vi "TxChannel - Get Tx Channels.vi"(7 "MCLB":refnum<vi>, 8 "error in (no error)":errorcluster, 11 "Node Ptr":T1 format="%.0x") -> (0 "error out":errorcluster, 3 "Node Ptr out":T1 format="%.0x", 5 "Channel Info":string[][](array[string]))   [LabVIEW 2019, in "UDP-Custom-Device System Explorer.lvlib"]
uses:
  UDP-Custom-Device System Explorer.lvlib
  <vilib>/NI VeriStand/Custom Device API/Custom Device Item Ref.ctl
  <vilib>/NI VeriStand/Custom Device API/Custom Device API.lvlib
  Shared/UDP-Custom-Device Shared.lvlib
  Property Accessors/Tx Channel Section Accessors.lvlib
  Property Accessors/Tx Channel Accessors.lvlib
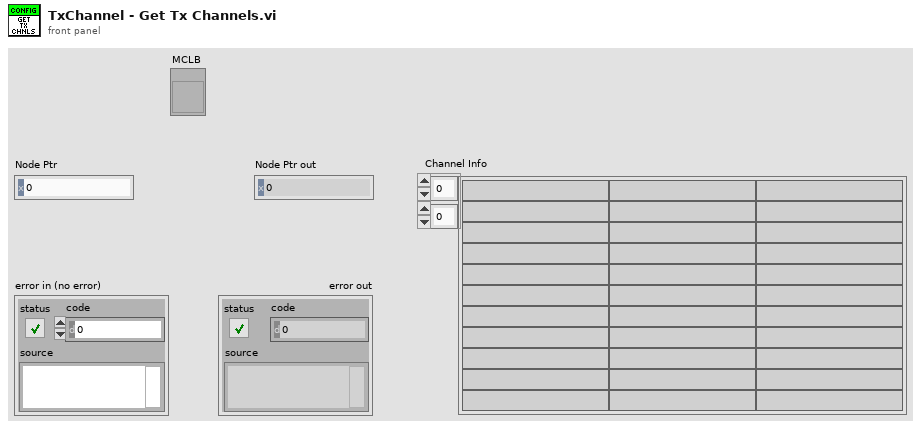
[diagram p1: front panel]
types:
  T1 = typedef "Custom Device API.lvlib/Custom Device Item Ref.ctl" = u64
  T2 = typedef "Custom Device API.lvlib/Custom Device Item Info.ctl" = cluster{"Name":string, "Is Channel":bool, "GUID":string, "Is Waveform":bool}
  T3 = typedef "UDP-Custom-Device Shared.lvlib/Shared - Channel Data Type.ctl" = enum16{"Boolean", "Single", "Double", "I8", "I16", "I32", "I64", "U8", "U16", "U32", "U64"}
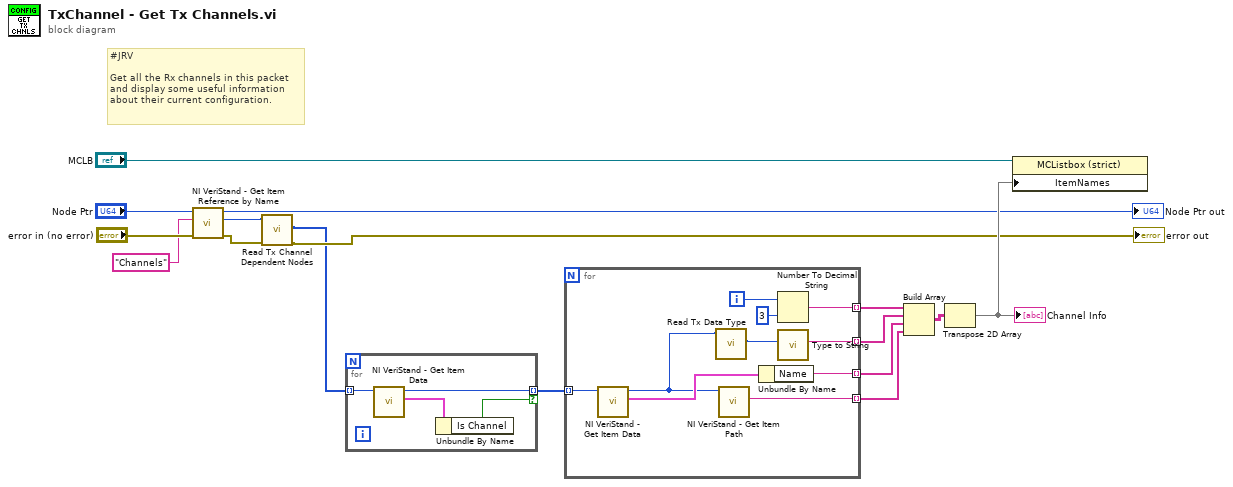
[diagram p0: block diagram]
diagram:
  # "#JRV\n\nGet all the Rx channels in this packet\nand display some useful information\nabout their current configuration."
  n1 = call <vilib>:"NI VeriStand - Get Item Reference by Name.vi"("error in (no error)"="error in (no error)", "Item Name"="Channels" ("Section Name"), "Parent Ref in"="Node Ptr") -> ("error out"=w5:errorcluster, "Item Ref"=w4:T1, "Parent Ref out"=→"Node Ptr out":T1)  [unwired: 5 in, 1 out]
  n2 = call "Read Tx Channel Dependent Nodes.vi"("error in (no error)"=w5, "Node Ptr"=w4) -> ("error out"=→"error out":errorcluster, "Dependent Node Refs"=w2:T1[])  [unwired: 7 in, 1 out]
  n3 = for {
    tunnel: [w19] -> w12 mode=indexing if=w17
    tunnel: w2 -> [w20] mode=indexing
    n4 = call <vilib>:"NI VeriStand - Get Item Data.vi"("Item Ref in"=w20) -> ("Item Info"=w18:T2, "Item Ref out"=w19:T1)  [unwired: 7 in, 2 out]
    n5 = Unbundle By Name(w18) -> ("Is Channel"=w17:bool)
  }
  n6 = for {
    tunnel: w12 -> [w30] mode=indexing
    tunnel: [w24] -> w8 mode=indexing
    tunnel: [w26] -> w7 mode=indexing
    tunnel: [w25] -> w16 mode=indexing
    tunnel: [w21] -> w1 mode=indexing
    i -> [w28]
    n7 = call <vilib>:"NI VeriStand - Get Item Data.vi"("Item Ref in"=w30) -> ("Item Info"=w29:T2, "Item Ref out"=w22:T1)  [unwired: 7 in, 2 out]
    n8 = call "Read Tx Data Type.vi"("Node Ptr"=w22) -> ("Data Type"=w23:T3)  [unwired: 7 in, 3 out]
    n9 = call <vilib>:"NI VeriStand - Get Item Path.vi"("Item Ref in"=w22) -> ("Path"=w21:string)  [unwired: 7 in, 3 out]
    n10 = Unbundle By Name(w29) -> ("Name"=w26:string)
    n11 = Number To Decimal String(number=w28, width (-)=i16 3) -> (decimal integer string=w25:string)
    n12 = call "Type to String.vi"("Data Type"=w23) -> ("String Type"=w24:string)  [unwired: 10 in]
  }
  n13 = Build Array(w16, w8, w7, w1) -> (w14:string[][])
  n14 = Transpose 2D Array(2D array=w14) -> (transposed array=w13:string[][])
  "Channel Info" <- w13
  n15 = property class="MCListbox (strict)"(reference="MCLB", "ItemNames"=w13) -> ()  [unwired: 1 in, 2 out]
